vi "Channel Count.vi"(8 "error in (no error)":errorcluster, 11 "Transfer Group Configuration in":refnum<class "Transfer Group Configuration.lvclass">) -> (0 "error out":errorcluster, 2 "total channel count":u64, 3 "Transfer Group Configuration out":refnum<class "Transfer Group Configuration.lvclass">)   [LabVIEW 2017, in "DSF Core.lvlib" / "Transfer Group Configuration.lvclass"]
uses:
  Transfer Group Configuration.lvclass
  Transfer Group Configuration.lvclass/Transfer Group Configuration.ctl
  Transfer/Transfer Configuration.lvclass
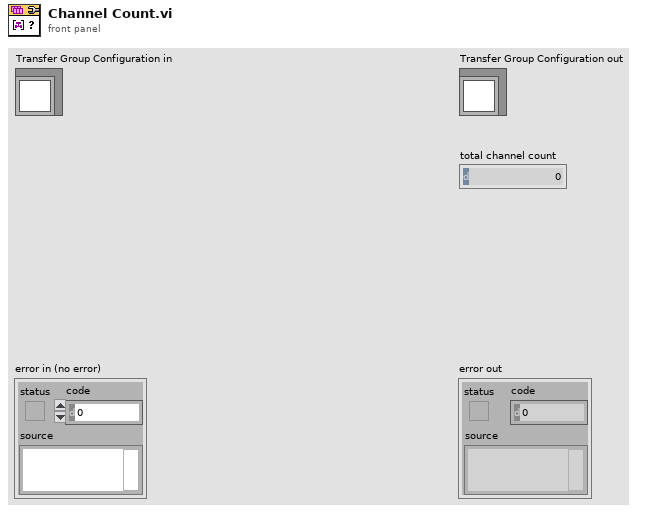
[diagram p1: front panel]
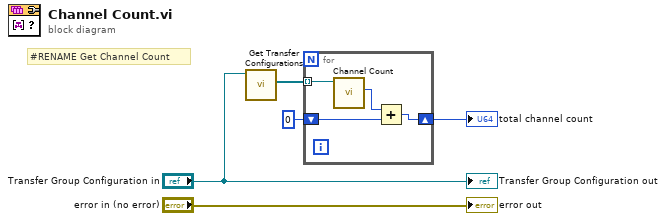
[diagram p0: block diagram]
diagram:
  # "#RENAME Get Channel Count"
  n1 = call "Get Transfer Configurations.vi"("Transfer Group Configuration in"="Transfer Group Configuration in") -> ("Transfer Configurations"=w4:refnum<class "Transfer Configuration.lvclass">[])  [unwired: 9 in, 1 out]
  n2 = for {
    tunnel: w4 -> [w7] mode=indexing
    shift-right: [w9] -> w1
    shift-left: u64 0 -> [w8]
    n3 = call "Channel Count.vi"("Transfer Configuration in"=w7) -> ("total channel count"=w6:u64)  [unwired: 8 in, 2 out]
    n4 = Add(x=w6, y=w8) -> (x+y=w9:u64)
  }
  "total channel count" <- w1
  "error out" <- "error in (no error)"
  "Transfer Group Configuration out" <- "Transfer Group Configuration in"
